vi "Get Full Name.vi"(7 "Include Extra Info":bool, 11 "CIFPluginLoader in":refnum<class "CIFPluginLoader.lvclass">) -> (3 "Name":string)   [LabVIEW 2021, in "CIFPluginLoader.lvclass"]
uses:
  CIFPluginLoader.lvclass
  CIFPluginLoader.lvclass/CIFPluginLoader.ctl
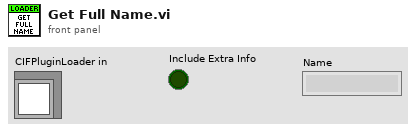
[diagram p1: front panel]
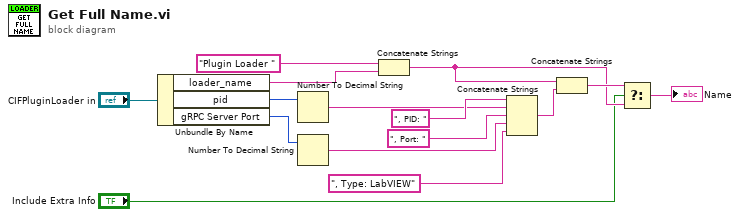
[diagram p0: block diagram]
diagram:
  n1 = Unbundle By Name("CIFPluginLoader in") -> ("loader_name"=w8:string, "pid"=w13:u32, "gRPC Server Port"=w11:i32)
  n2 = Number To Decimal String(number=w13) -> (decimal integer string=w14:string)  [unwired: 1 in]
  n3 = Number To Decimal String(number=w11) -> (decimal integer string=w10:string)  [unwired: 1 in]
  n4 = Concatenate Strings("Plugin Loader " ("message"), w8) -> (w3:string)
  n5 = Concatenate Strings(", PID: " ("message"), w14, ", Port: " ("message"), w10, ", Type: LabVIEW" ("message")) -> (w5:string)
  n6 = Concatenate Strings(w3, w5) -> (w4:string)
  n7 = Select(t=w4, s="Include Extra Info", f=w3) -> (s? t:f=→"Name":string)
